vi "STS_Get_Mueller_Raw_Data.vi"(8 "错误输入（无错误）":errorcluster, 11 ".NET引用句柄输入":refnum<k24>) -> (0 "error out":errorcluster, 3 "引用输出":refnum<k24>, 4 "m14":dbl[](array[numeric]), 5 "m12":dbl[](array[numeric]), 6 "m13":dbl[](array[numeric]), 7 "m11":dbl[](array[numeric]))   [LabVIEW 2017]
doc: "Process ranges merge"
uses:
  D:/test/PDLSTS/LV_PDL_Sample/DLL/STSProcess.dll
  DLL/STSProcess.dll
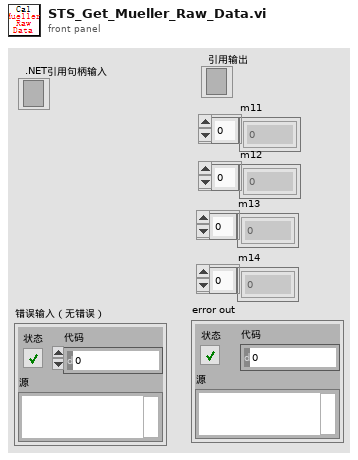
[diagram p1: front panel]
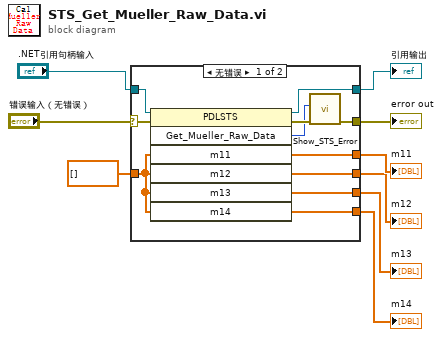
[diagram p0: block diagram]
diagram:
  n1 = case shown="无错误" "错误输入（无错误）" {
    selector: "错误输入（无错误）" -> [w19 w23]
    tunnel: ".NET引用句柄输入" -> [w20 w22]
    tunnel: [w16 w23] -> w7
    tunnel: [w15 w22] -> w6
    tunnel: dbl[] [] ("m11") -> [w14 w21]
    tunnel: [w13 w21] -> w4
    tunnel: [w12 w21] -> w3
    tunnel: [w11 w21] -> w2
    tunnel: [w10 w21] -> w1
    frame No Error {
      n2 = invoke class="PDLSTS" method="Get_Mueller_Raw_Data"(reference=w20, error in=w19, "m11"=w14, "m12"=w14, "m13"=w14, "m14"=w14) -> (reference out=w15:refnum<k24>, error out=w18:errorcluster, "Get_Mueller_Raw_Data"=w17:i32, "m11"=w13:dbl[], "m12"=w12:dbl[], "m13"=w11:dbl[], "m14"=w10:dbl[])  [unwired: 1 in]
      n3 = call "Show_STS_Error.vi"("error in (no error)"=w18, "Error"=w17) -> ("error out"=w16:errorcluster)  [unwired: 9 in]
    }
    frame Error {
    }
  }
  "error out" <- w7
  "引用输出" <- w6
  "m11" <- w4
  "m12" <- w3
  "m13" <- w2
  "m14" <- w1
